vi "Release.vi"(8 "Error In":errorcluster, 11 "Listeners In":refnum<queue>[](array[refnum])) -> (0 "Error Out":errorcluster, 3 "Listeners Out":refnum<queue>[](array[refnum]))   [LabVIEW 2018, in "Toolkit.lvlib"]
uses:
  Toolkit.lvlib
  Type Definitions/Statement.ctl
  Type Definitions/Tag.ctl
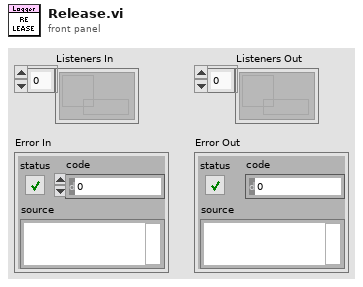
[diagram p1: front panel]
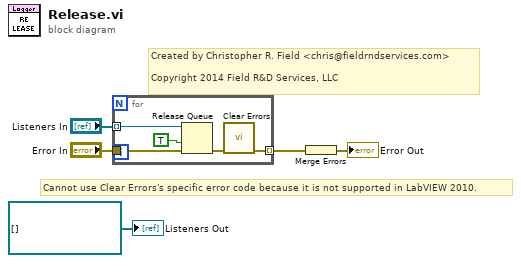
[diagram p0: block diagram]
diagram:
  # "Cannot use Clear Errors's specific error code because it is not supported in LabVIEW 2010."
  # "Created by Christopher R. Field <chris@fieldrndservices.com>\n\nCopyright 2014 Field R&D Services, LLC"
  n1 = for {
    tunnel: "Listeners In" -> [w10] mode=indexing
    tunnel: "Error In" -> [w9]
    tunnel: [w6] -> w1 mode=indexing
    n2 = Release Queue(queue=w10, force destroy? (F)=TRUE, error in (no error)=w9) -> (error out=w7:errorcluster)  [unwired: 2 out]
    n3 = call <vilib>:"Clear Errors.vi"("error in (no error)"=w7) -> ("error out"=w6:errorcluster)  [unwired: 5 in, 1 out]
  }
  n4 = Merge Errors(w1) -> (→"Error Out":errorcluster)
  "Listeners Out" <- refnum<queue>[] [] ("Listeners Out")
